vi "rx metadata has time spec.vi"(8 "error in (no error)":errorcluster, 10 "result_out":i32, 11 "h":u64) -> (0 "error out":errorcluster, 1 "function return":u32(ring), 2 "result_out out":i32, 3 "h out":u64)   [LabVIEW 2023, in "uhd.lvlib"]
doc: "UHD_API uhd_error uhd_rx_metadata_has_time_spec(\n uhd_rx_metadata_handle h, bool* result_out);"
uses:
  <userlib>/uhd/uhd.lvlib
  <userlib>/uhd/uhd.dll
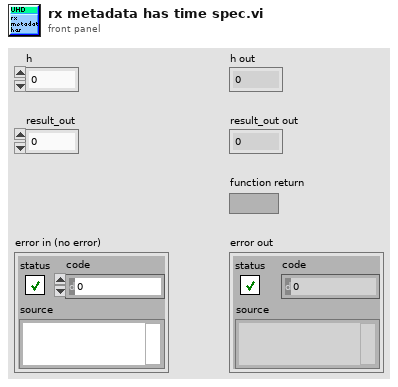
[diagram p1: front panel]
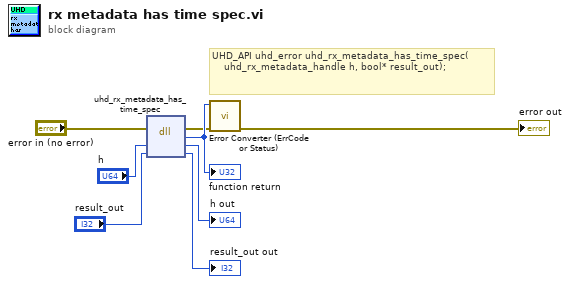
[diagram p0: block diagram]
diagram:
  # "UHD_API uhd_error uhd_rx_metadata_has_time_spec(\n    uhd_rx_metadata_handle h, bool* result_out);"
  n1 = dll-call lib="C:/Program Files/National Instruments/LabVIEW 2023/user.lib/uhd/uhd.*" fn="uhd_rx_metadata_has_time_spec"(error in="error in (no error)", "h"="h", "result_out"="result_out") -> (error out=w2:errorcluster, w8:u32, "h"=→"h out":u64, "result_out"=→"result_out out":i32)  [unwired: 2 in, 1 out]
  "function return" <- w8
  n2 = call <userlib>:"Error Converter (ErrCode or Status).vi"("error in (no error)"=w2, "error code"=w8) -> ("error out"=→"error out":errorcluster)  [unwired: 9 in]
